vi "bob1tobun.vi"() -> ()   [LabVIEW 2014, in "Panels.lvlib"]
uses:
  Panels.lvlib
  CSlibraries-extern/DimLVEvent/DimIndicators/DimIndicators.lvlib
  CSlibraries/UtilityLib/UtilityLib.lvlib
  CS_Core/CSSystem/CoreLib/CoreLib.lvlib
  CSlibraries/UtilityLib/UtilityLib.valueStatus.ctl
  CSlibraries-extern/DimLVEvent/LVDimInterface/LVDimInterface.lvlib
  Instance           1 17Saved   bob1tobun .vi
  CSlibraries-extern/DimLVEvent/DimIndicators/DimIndicators.numericArrayType.ctl
  CSlibraries-extern/DimLVEvent/DimIndicators/DimIndicators.anyType.ctl
  CSlibraries-extern/DimLVEvent/DimIndicators/DimIndicators.numericType.ctl
panel:
  out "DIM Error":bool
  in  "SetFileLocation_Data":T1={"data"="NOLINK", "no link"=TRUE, "quality"=-1, "timeStamp"=0.0}
  in  "Q90PlanDefY":bool
  in  "ISDefY":bool
  in  "Q90PlanLens":bool
  in  "BOB3DefY":bool
  in  "BOB3DefX":bool
  in  "BOB2Q90Lens":bool
  in  "Q90DefMain":bool
  in  "Q90BOB3Lens":bool
  in  "ISDefX":bool
  in  "Q90CylLens":bool
  in  "BOB2DefX":bool
  in  "BOB2DefY":bool
  in  "WalLens":bool
  in  "BOB1DefX":bool
  in  "BOB1DefY":bool
  in  "Q90DefMain_MonData":T2={"data"=inf, "no link"=FALSE, "quality"=1, "timeStamp"=3265900746.554}
  in  "Q90BOB3Lens_MonData":T2={"data"=inf, "no link"=FALSE, "quality"=1, "timeStamp"=3265900746.538}
  in  "Q90PlanLens_MonData":T2={"data"=inf, "no link"=FALSE, "quality"=1, "timeStamp"=3265900746.522}
  in  "BOB3DefX_MonData":T2={"data"=inf, "no link"=FALSE, "quality"=1, "timeStamp"=3265900746.554}
  in  "BOB1DefX_MonData":T2={"data"=inf, "no link"=FALSE, "quality"=1, "timeStamp"=3265900746.538}
  in  "WalLens_MonData":T2={"data"=inf, "no link"=FALSE, "quality"=1, "timeStamp"=3265900746.569}
  in  "BOB2Q90Lens_MonData":T2={"data"=inf, "no link"=FALSE, "quality"=1, "timeStamp"=3265900746.554}
  in  "ISDefX_MonData":T2={"data"=inf, "no link"=FALSE, "quality"=1, "timeStamp"=3265900746.538}
  in  "BOB2DefX_MonData":T2={"data"=inf, "no link"=FALSE, "quality"=1, "timeStamp"=3265900746.569}
  in  "BOB3DefY_MonData":T2={"data"=inf, "no link"=FALSE, "quality"=1, "timeStamp"=3265900746.569}
  in  "Q90DefCorr1_MonData":T2={"data"=inf, "no link"=FALSE, "quality"=1, "timeStamp"=3265900746.538}
  in  "Q90DefCorr2_MonData":T2={"data"=inf, "no link"=FALSE, "quality"=1, "timeStamp"=3265900746.585}
  in  "Q90PlanDefY_MonData":T2={"data"=inf, "no link"=FALSE, "quality"=1, "timeStamp"=3265900746.538}
  in  "Q90DefMain1_MonData":T2={"data"=inf, "no link"=FALSE, "quality"=1, "timeStamp"=3265900746.554}
  in  "ISDefY_MonData":T2={"data"=inf, "no link"=FALSE, "quality"=1, "timeStamp"=3265900746.522}
  in  "BOB1DefY_MonData":T2={"data"=inf, "no link"=FALSE, "quality"=1, "timeStamp"=3265900746.538}
  in  "BOB2DefY_MonData":T2={"data"=inf, "no link"=FALSE, "quality"=1, "timeStamp"=3265900746.6}
  in  "Q90CylLens_MonData":T2={"data"=inf, "no link"=FALSE, "quality"=1, "timeStamp"=3265900746.585}
  in  "Q90DefMain2_MonData":T2={"data"=inf, "no link"=FALSE, "quality"=1, "timeStamp"=3265900746.569}
  in  "Q90DefMain_SetValueInfoData":T3={"data"=[-400.0, 400.0, 3.0], "no link"=FALSE, "quality"=0, "timeStamp"=3265900746.554}
  in  "Q90DefMain_SetData":T3={"data"=[0.0, 0.0, 0.0, 0.0], "no link"=FALSE, "quality"=1, "timeStamp"=3265900745.1}
  out "Q90DefMain_Mon":dbl=inf format="%.4f"
  in  "BOB1DefX_SetValueInfoData":T3={"data"=[-404.0, 401.8, 3.0], "no link"=FALSE, "quality"=0, "timeStamp"=3265900746.569}
  in  "BOB1DefX_SetData":T3={"data"=[0.0, 0.0, 0.0, 0.0], "no link"=FALSE, "quality"=1, "timeStamp"=3265900745.053}
  out "BOB3DefX_Mon":dbl=inf format="%.4f"
  in  "BOB1DefY_SetData":T3={"data"=[0.0, 0.0, 0.0, 0.0], "no link"=FALSE, "quality"=1, "timeStamp"=3265900745.053}
  in  "BOB3DefY_SetValueInfoData":T3={"data"=[-400.0, 400.0, 3.0], "no link"=FALSE, "quality"=0, "timeStamp"=3265900746.554}
  in  "BOB3DefX_SetValueInfoData":T3={"data"=[-400.0, 400.0, 3.0], "no link"=FALSE, "quality"=0, "timeStamp"=3265900746.538}
  in  "Q90BOB3Lens_SetValueInfoData":T3={"data"=[-400.0, 400.0, 3.0], "no link"=FALSE, "quality"=0, "timeStamp"=3265900746.522}
  in  "ISDefY_SetValueInfoData":T3={"data"=[-118.7, 118.8, 3.0], "no link"=FALSE, "quality"=0, "timeStamp"=3265900746.569}
  in  "Q90PlanDefY_SetValueInfoData":T3={"data"=[-120.9, 120.5, 3.0], "no link"=FALSE, "quality"=0, "timeStamp"=3265900746.585}
  in  "Q90PlanLens_SetValueInfoData":T3={"data"=[-120.8, 120.3, 3.0], "no link"=FALSE, "quality"=0, "timeStamp"=3265900746.569}
  in  "BOB3DefY_SetData":T3={"data"=[0.0, 0.0, 0.0, 0.0], "no link"=FALSE, "quality"=1, "timeStamp"=3265900745.1}
  in  "BOB3DefX_SetData":T3={"data"=[0.0, 0.0, 0.0, 0.0], "no link"=FALSE, "quality"=1, "timeStamp"=3265900745.085}
  in  "Q90BOB3Lens_SetData":T3={"data"=[0.0, 0.0, 0.0, 0.0], "no link"=FALSE, "quality"=1, "timeStamp"=3265900745.069}
  in  "ISDefY_SetData":T3={"data"=[0.0, 0.0, 0.0, 0.0], "no link"=FALSE, "quality"=1, "timeStamp"=3265900745.069}
  in  "Q90PlanDefY_SetData":T3={"data"=[0.0, 0.0, 0.0, 0.0], "no link"=FALSE, "quality"=1, "timeStamp"=3265900745.069}
  out "Q90PlanLens_Mon":dbl=inf format="%.4f"
  out "Q90BOB3Lens_Mon":dbl=inf format="%.4f"
  out "BOB3DefY_Mon":dbl=inf format="%.4f"
  out "Q90DefMain1_Mon":dbl=inf format="%.4f"
  out "Q90DefCorr2_Mon":dbl=inf format="%.4f"
  out "Q90DefCorr1_Mon":dbl=inf format="%.4f"
  out "Q90PlanDefY_Mon":dbl=inf format="%.4f"
  in  "Q90PlanLens_SetData":T3={"data"=[0.0, 0.0, 0.0, 0.0], "no link"=FALSE, "quality"=1, "timeStamp"=3265900745.069}
  out "WalLens_Mon":dbl=inf format="%.4f"
  out "BOB1DefX_Mon":dbl=inf format="%.4f"
  out "i ref out":refnum<vi>
  in  "Last Loaded File_Data":T1={"data"="NOLINK", "no link"=TRUE, "quality"=-1, "timeStamp"=0.0}
  out "FileUpToDate":bool=TRUE caption="Parameter Changed"
  in  "Close All Panels":bool
  in  "WalLens_SetValueInfoData":T3={"data"=[-401.3, 400.4, 3.0], "no link"=FALSE, "quality"=0, "timeStamp"=3265900746.554}
  in  "BOB2Q90Lens_SetValueInfoData":T3={"data"=[-404.3, 403.0, 3.0], "no link"=FALSE, "quality"=0, "timeStamp"=3265900746.538}
  in  "BOB2DefX_SetValueInfoData":T3={"data"=[-400.3, 399.3, 3.0], "no link"=FALSE, "quality"=0, "timeStamp"=3265900746.569}
  in  "BOB2DefY_SetValueInfoData":T3={"data"=[0.0, 3000.0, -1.0], "no link"=FALSE, "quality"=0, "timeStamp"=3265900746.554}
  in  "Q90CylLens_SetValueInfoData":T3={"data"=[0.0, 1500.0, -1.0], "no link"=FALSE, "quality"=0, "timeStamp"=3265900746.554}
  in  "ISDefX_SetValueInfoData":T3={"data"=[0.0, 1000.0, -1.0], "no link"=FALSE, "quality"=0, "timeStamp"=3265900746.538}
  in  "BOB1DefY_SetValueInfoData":T3={"data"=[-404.0, 401.8, 3.0], "no link"=FALSE, "quality"=0, "timeStamp"=3265900746.569}
  in  "ISDefX_SetData":T3={"data"=[0.0, 0.0, 0.0, 0.0], "no link"=FALSE, "quality"=1, "timeStamp"=3265900745.069}
  in  "Q90CylLens_SetData":T3={"data"=[0.0, 0.0, 0.0, 0.0], "no link"=FALSE, "quality"=1, "timeStamp"=3265900745.053}
  in  "BOB2DefY_SetData":T3={"data"=[0.0, 0.0, 0.0, 0.0], "no link"=FALSE, "quality"=1, "timeStamp"=3265900745.085}
  in  "BOB2DefX_SetData":T3={"data"=[0.0, 0.0, 0.0, 0.0], "no link"=FALSE, "quality"=1, "timeStamp"=3265900745.085}
  in  "BOB2Q90Lens_SetData":T3={"data"=[0.0, 0.0, 0.0, 0.0], "no link"=FALSE, "quality"=1, "timeStamp"=3265900745.085}
  in  "WalLens_SetData":T3={"data"=[0.0, 0.0, 0.0, 0.0], "no link"=FALSE, "quality"=1, "timeStamp"=3265900745.053}
  out "Last Loaded File":string
  in  "SetFileLocation":path=path "\\\\intranet\\Files/projects/lebit/Data Exchange/data/bob1tobunControl"
  out "ISDefY_Mon":dbl=inf format="%.4f"
  out "Q90CylLens_Mon":dbl=inf format="%.4f"
  out "BOB1DefY_Mon":dbl=inf format="%.4f"
  out "BOB2DefY_Mon":dbl=inf format="%.4f"
  out "Q90DefMain2_Mon":dbl=inf format="%.4f"
  out "BOB2DefX_Mon":dbl=inf format="%.4f"
  out "ISDefX_Mon":dbl=inf format="%.4f"
  out "BOB2Q90Lens_Mon":dbl=inf format="%.4f"
  # "Parameter changed, data file is no longer up-to-date."
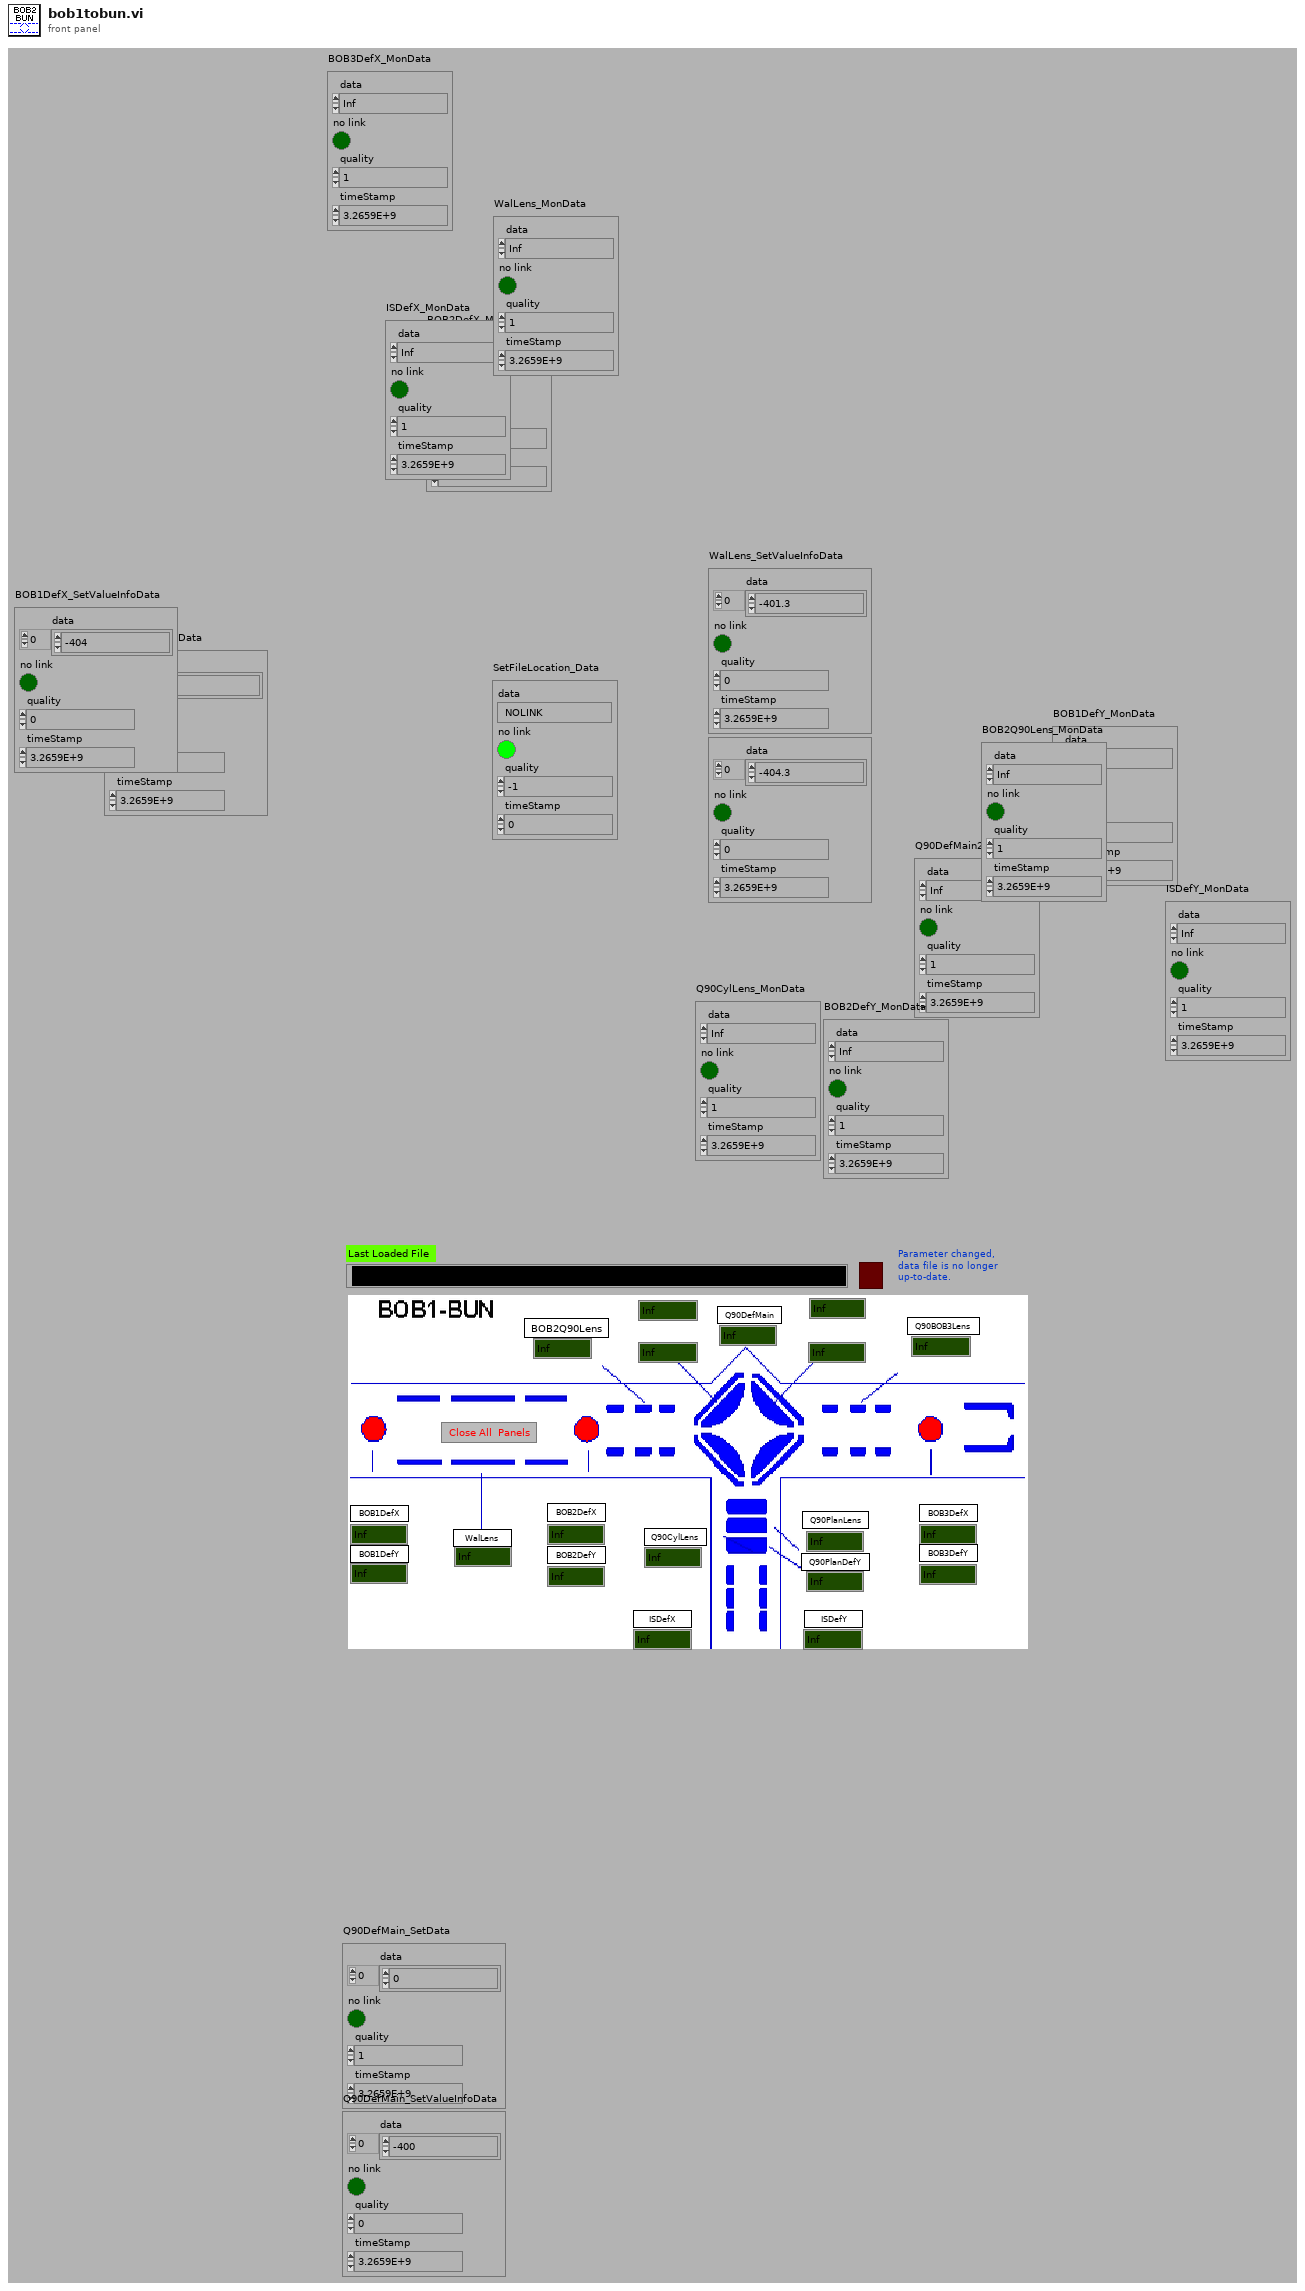
[diagram p1: front panel]
types:
  T1 = typedef "DimIndicators.lvlib/DimIndicators.anyType.ctl" = cluster{"data":string, "no link":bool, "quality":i32, "timeStamp":dbl}
  T2 = typedef "DimIndicators.lvlib/DimIndicators.numericType.ctl" = cluster{"data":dbl, "no link":bool, "quality":i32, "timeStamp":dbl}
  T3 = typedef "DimIndicators.lvlib/DimIndicators.numericArrayType.ctl" = cluster{"data":dbl[], "no link":bool, "quality":i32, "timeStamp":dbl}
  T4 = typedef "UtilityLib.lvlib/UtilityLib.valueStatus.ctl" = enum16{"no info available", "stand by/off", "on", "warning", "alarm/malfunction", "not implemented", "user action required", "important information", "system default", "control default", "indicator default", "button default"}
  T5 = cluster{"data":string, "no link":bool, "quality":i32, "timeStamp":dbl}
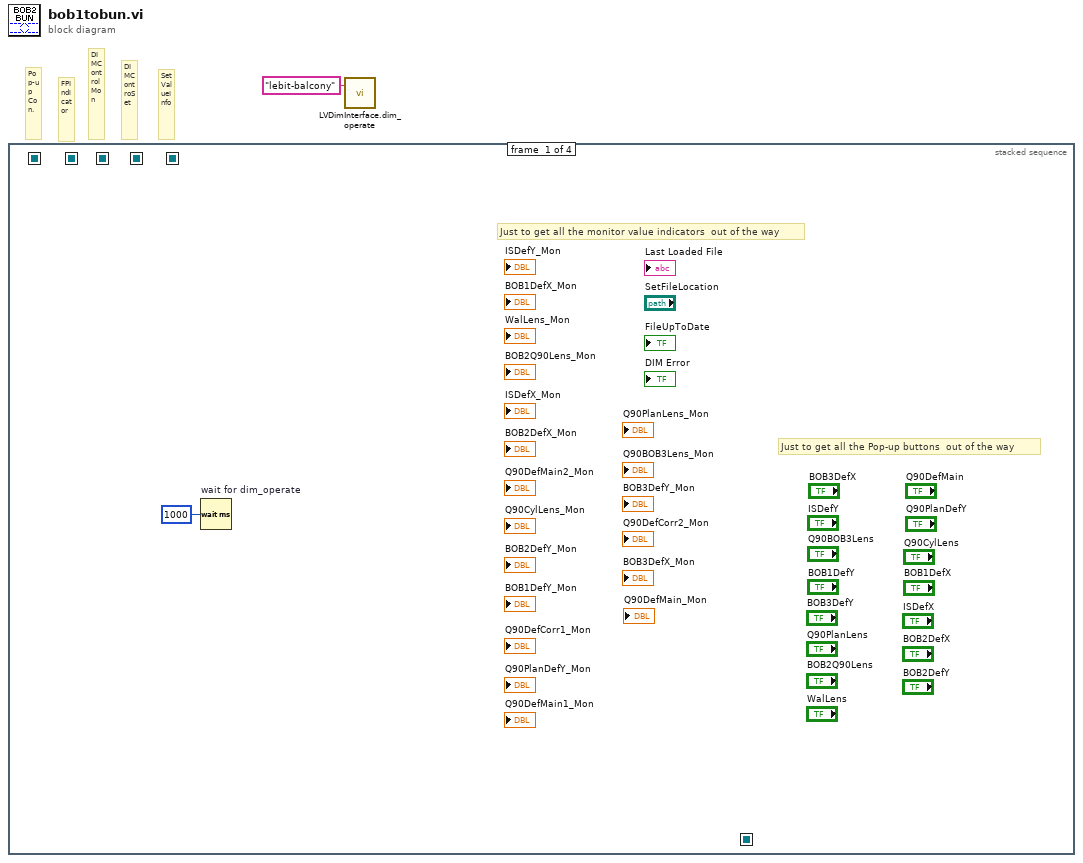
[diagram p0: block diagram]
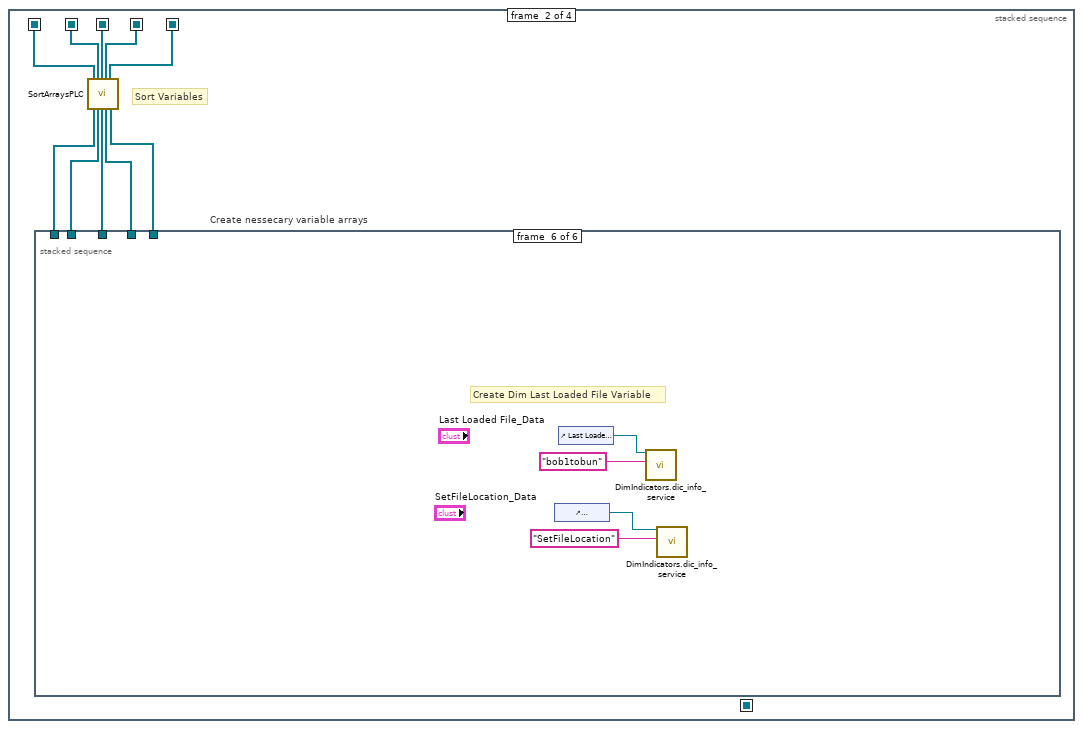
[diagram p2: hidden frame]
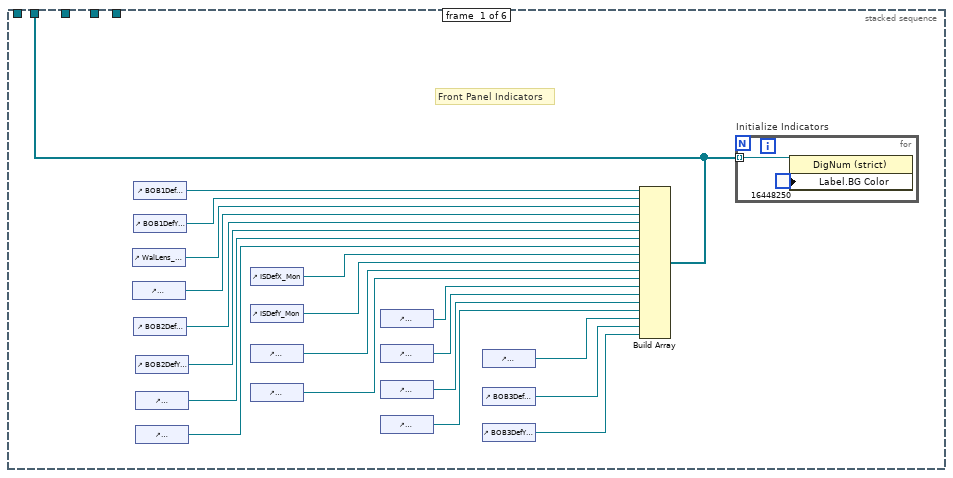
[diagram p3: hidden frame]
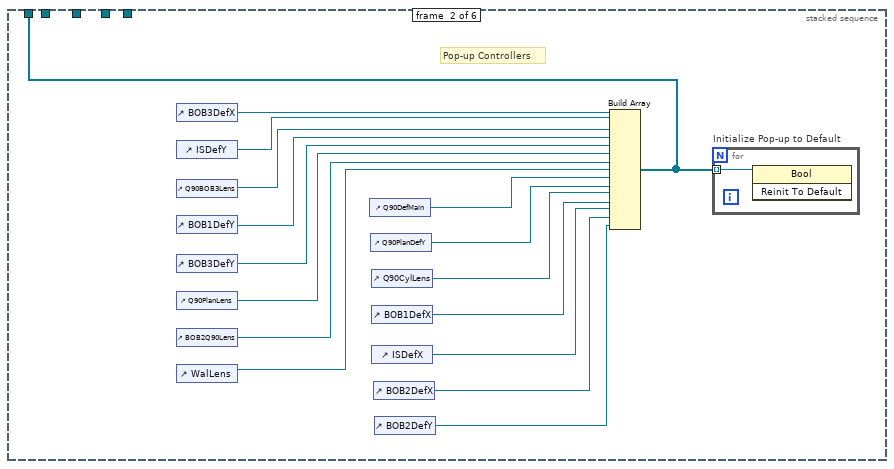
[diagram p4: hidden frame]
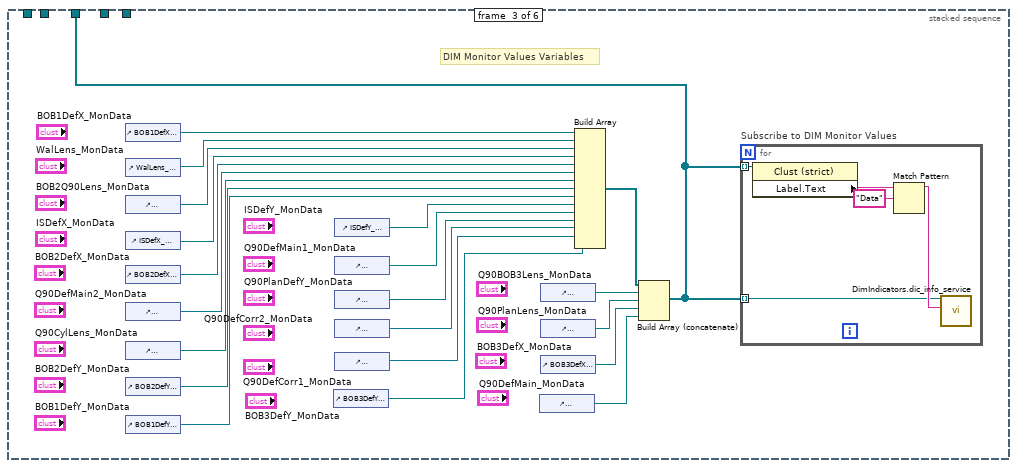
[diagram p5: hidden frame]
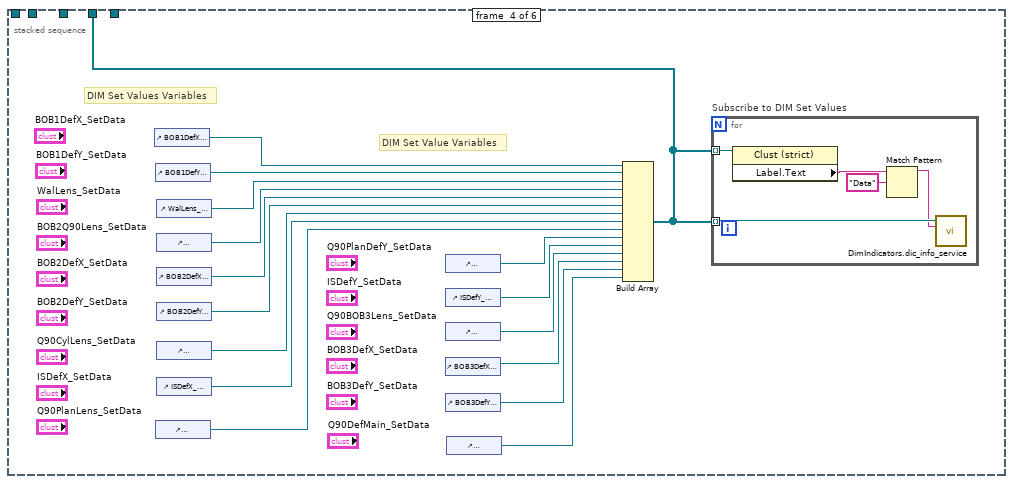
[diagram p6: hidden frame]
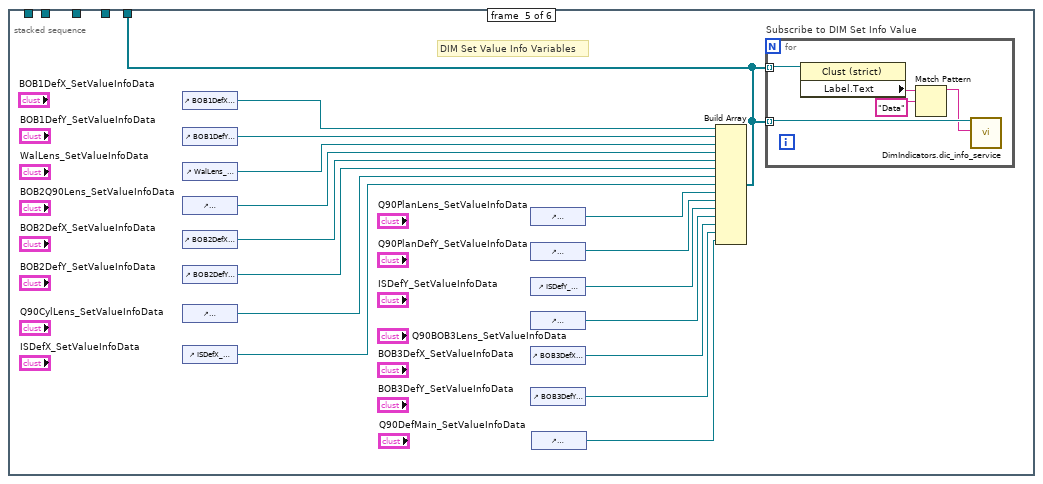
[diagram p7: hidden frame]
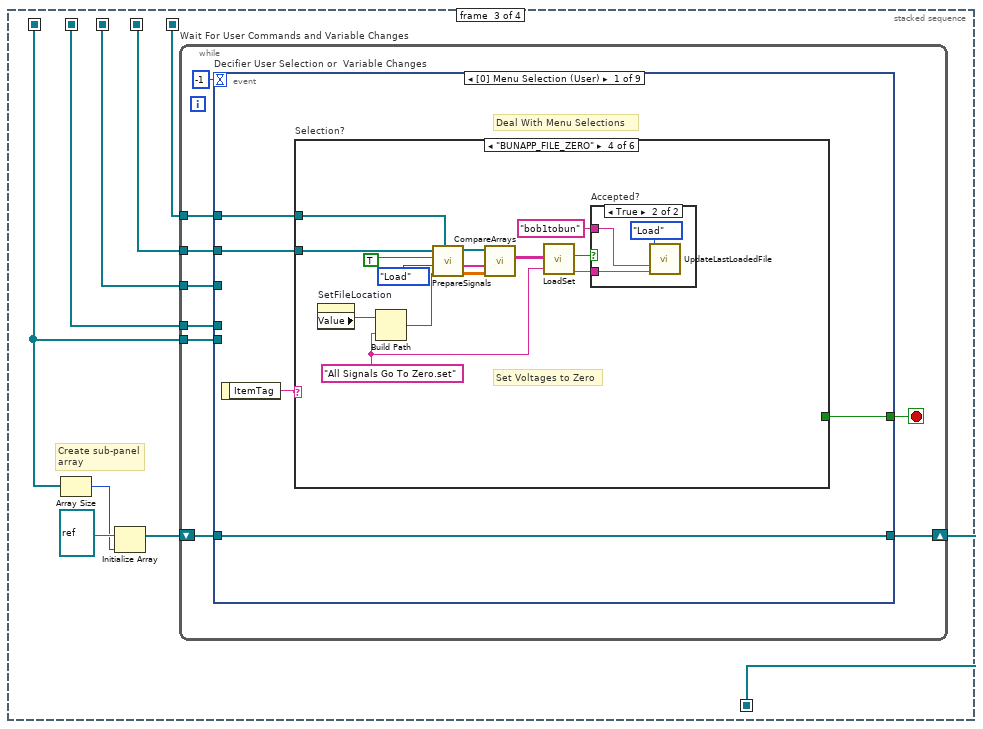
[diagram p8: hidden frame]
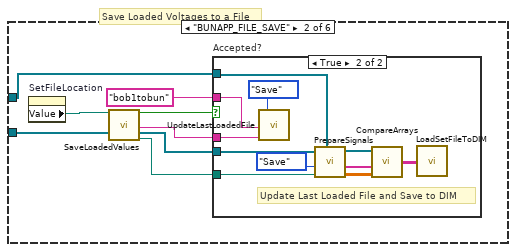
[diagram p10: hidden frame]
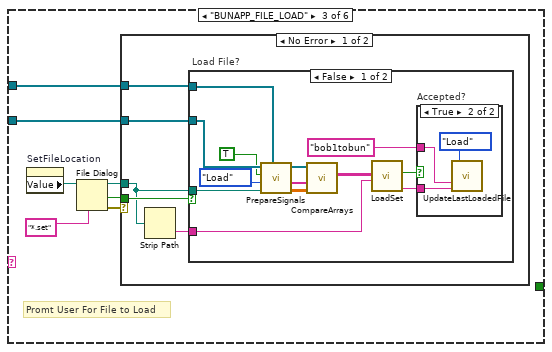
[diagram p12: hidden frame]
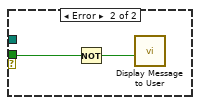
[diagram p15: hidden frame]
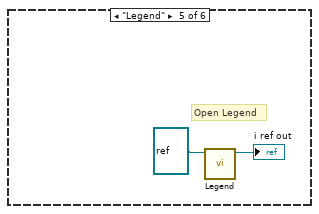
[diagram p17: hidden frame]
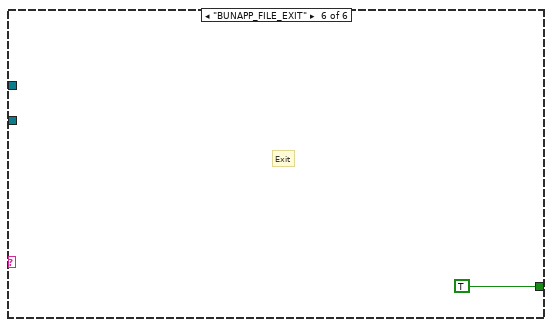
[diagram p18: hidden frame]
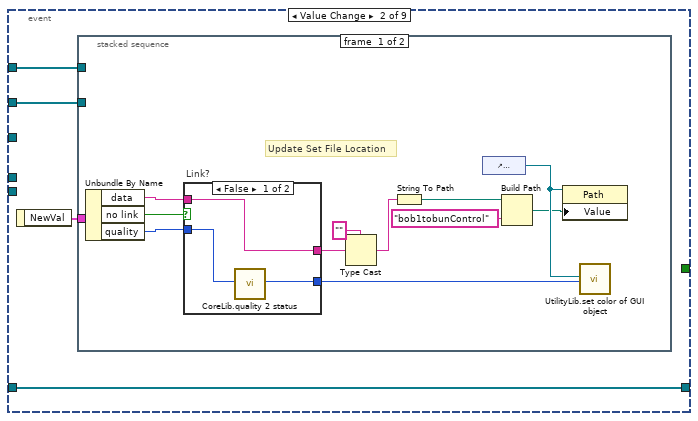
[diagram p19: hidden frame]
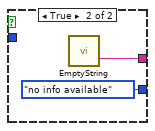
[diagram p20: hidden frame]
diagram:
  # "Pop-up Con."
  # "SetValueInfo"
  # "DIMControSet"
  # "DIMControlMon"
  # "FPIndicator"
  n1 = stacked-sequence {
    seq-local: [_ w4 _ _] -> [_ _ w130 _]
    seq-local: [_ w5 _ _] -> [_ _ w125 w325]
    seq-local: [_ _ w128 _] -> [_ _ _ w324]
    seq-local: [_ w6 _ _] -> [_ _ w127 w323]
    seq-local: [_ w7 _ _] -> [_ _ w126 w322]
    seq-local: [_ w3 _ _] -> [_ _ w124 _]
    frame #0 {
      # "Just to get all the Pop-up buttons  out of the way"
      # "Just to get all the monitor value indicators  out of the way"
      n2 = Wait (ms) "wait for dim_operate"(milliseconds to wait=u32 1000) -> ()  [unwired: 1 out]
    }
    frame #1 {
      # "Sort Variables"
      # "Arrange references to all monitor-value related buttons into an array."
      n3 = stacked-sequence "Create nessecary variable arrays" {
        tunnel: [w31 _ _ _ _ _] -> w11
        tunnel: [_ w35 _ _ _ _] -> w12
        tunnel: [_ _ w52 _ _ _] -> w10
        tunnel: [_ _ _ w78 _ _] -> w9
        tunnel: [_ _ _ _ w99 _] -> w8
        frame #0 {
          # "Front Panel Indicators"
          n4 = control-ref of="WalLens_Mon"() -> (w24:refnum<vi>)
          n5 = control-ref of="BOB2Q90Lens_Mon"() -> (w23:refnum<vi>)
          n6 = control-ref of="BOB1DefX_Mon"() -> (w30:refnum<vi>)
          n7 = control-ref of="BOB1DefY_Mon"() -> (w25:refnum<vi>)
          n8 = control-ref of="BOB2DefX_Mon"() -> (w32:refnum<vi>)
          n9 = control-ref of="BOB2DefY_Mon"() -> (w21:refnum<vi>)
          n10 = control-ref of="Q90DefMain2_Mon"() -> (w20:refnum<vi>)
          n11 = control-ref of="Q90CylLens_Mon"() -> (w19:refnum<vi>)
          n12 = control-ref of="ISDefX_Mon"() -> (w22:refnum<vi>)
          n13 = control-ref of="ISDefY_Mon"() -> (w29:refnum<vi>)
          n14 = control-ref of="Q90DefMain_Mon"() -> (w17:refnum<vi>)
          n15 = control-ref of="Q90DefMain1_Mon"() -> (w16:refnum<vi>)
          n16 = control-ref of="Q90DefCorr2_Mon"() -> (w28:refnum<vi>)
          n17 = control-ref of="Q90DefCorr1_Mon"() -> (w27:refnum<vi>)
          n18 = control-ref of="Q90PlanLens_Mon"() -> (w15:refnum<vi>)
          n19 = control-ref of="Q90PlanDefY_Mon"() -> (w14:refnum<vi>)
          n20 = control-ref of="Q90BOB3Lens_Mon"() -> (w13:refnum<vi>)
          n21 = control-ref of="BOB3DefX_Mon"() -> (w26:refnum<vi>)
          n22 = control-ref of="BOB3DefY_Mon"() -> (w18:refnum<vi>)
          n23 = Build Array(w30, w25, w24, w23, w32, w21, w20, w19, w22, w29, w17, w16, w28, w27, w15, w14, w13, w26, w18) -> (w31:refnum<vi>[])
          n24 = for "Initialize Indicators" {
            tunnel: w31 -> [w34] mode=indexing
            n25 = property class="DigNum (strict)"(reference=w34, "Label.BG Color"=u32 16448250 ("Color Box")) -> ()  [unwired: 1 in, 2 out]
          }
        }
        frame #1 {
          # "Pop-up Controllers"
          n26 = control-ref of="BOB3DefX"() -> (w50:refnum<vi>)
          n27 = control-ref of="ISDefY"() -> (w49:refnum<vi>)
          n28 = control-ref of="Q90BOB3Lens"() -> (w48:refnum<vi>)
          n29 = control-ref of="BOB1DefY"() -> (w47:refnum<vi>)
          n30 = control-ref of="BOB3DefY"() -> (w46:refnum<vi>)
          n31 = control-ref of="Q90PlanLens"() -> (w45:refnum<vi>)
          n32 = control-ref of="BOB2Q90Lens"() -> (w44:refnum<vi>)
          n33 = control-ref of="WalLens"() -> (w43:refnum<vi>)
          n34 = control-ref of="Q90DefMain"() -> (w42:refnum<vi>)
          n35 = control-ref of="Q90PlanDefY"() -> (w41:refnum<vi>)
          n36 = control-ref of="Q90CylLens"() -> (w40:refnum<vi>)
          n37 = control-ref of="BOB1DefX"() -> (w39:refnum<vi>)
          n38 = control-ref of="ISDefX"() -> (w38:refnum<vi>)
          n39 = control-ref of="BOB2DefX"() -> (w37:refnum<vi>)
          n40 = control-ref of="BOB2DefY"() -> (w36:refnum<vi>)
          n41 = Build Array(w50, w49, w48, w47, w46, w45, w44, w43, w42, w41, w40, w39, w38, w37, w36) -> (w35:refnum<vi>[])
          n42 = for "Initialize Pop-up to Default" {
            tunnel: w35 -> [w51] mode=indexing
            n43 = invoke class="Bool" method="Reinit To Default"(reference=w51) -> ()  [unwired: 2 in, 3 out]
          }
        }
        frame #2 {
          # "DIM Monitor Values Variables"
          n44 = control-ref of="BOB1DefX_MonData"() -> (w68:refnum<vi>)
          n45 = control-ref of="WalLens_MonData"() -> (w67:refnum<vi>)
          n46 = control-ref of="BOB2Q90Lens_MonData"() -> (w66:refnum<vi>)
          n47 = control-ref of="ISDefX_MonData"() -> (w61:refnum<vi>)
          n48 = control-ref of="BOB2DefX_MonData"() -> (w62:refnum<vi>)
          n49 = control-ref of="Q90DefMain2_MonData"() -> (w54:refnum<vi>)
          n50 = control-ref of="Q90CylLens_MonData"() -> (w55:refnum<vi>)
          n51 = control-ref of="BOB2DefY_MonData"() -> (w56:refnum<vi>)
          n52 = control-ref of="BOB1DefY_MonData"() -> (w57:refnum<vi>)
          n53 = control-ref of="BOB3DefY_MonData"() -> (w53:refnum<vi>)
          n54 = control-ref of="ISDefY_MonData"() -> (w58:refnum<vi>)
          n55 = control-ref of="Q90DefMain1_MonData"() -> (w59:refnum<vi>)
          n56 = control-ref of="Q90PlanDefY_MonData"() -> (w60:refnum<vi>)
          n57 = control-ref of="Q90DefCorr2_MonData"() -> (w69:refnum<vi>)
          n58 = control-ref of="Q90DefCorr1_MonData"() -> (w70:refnum<vi>)
          n59 = control-ref of="Q90DefMain_MonData"() -> (w72:refnum<vi>)
          n60 = control-ref of="Q90BOB3Lens_MonData"() -> (w63:refnum<vi>)
          n61 = control-ref of="Q90PlanLens_MonData"() -> (w64:refnum<vi>)
          n62 = control-ref of="BOB3DefX_MonData"() -> (w65:refnum<vi>)
          n63 = Build Array(w68, w67, w66, w61, w62, w54, w55, w56, w57, w58, w59, w60, w69, w70, w53) -> (w71:refnum<vi>[])
          n64 = Build Array (concatenate)(w71, w63, w64, w65, w72) -> (w52:refnum<vi>[])
          n65 = for "Subscribe to DIM Monitor Values" {
            tunnel: w52 -> [w74] mode=indexing
            tunnel: w52 -> [w73] mode=indexing
            n66 = property class="Clust (strict)"(reference=w73) -> ("Label.Text"=w76:string)  [unwired: 1 in, 2 out]
            n67 = Match Pattern(string=w76, regular expression="Data") -> (before substring=w75:string)  [unwired: 1 in, 3 out]
            n68 = call "DimIndicators.dic_info_service.vi"("controlRef"=w74, "serviceName"=w75) -> ()  [unwired: 16 in, 2 out]
          }
        }
        frame #3 {
          # "DIM Set Value Variables"
          # "DIM Set Values Variables"
          n69 = control-ref of="BOB1DefX_SetData"() -> (w80:refnum<vi>)
          n70 = control-ref of="BOB1DefY_SetData"() -> (w81:refnum<vi>)
          n71 = control-ref of="Q90PlanLens_SetData"() -> (w87:refnum<vi>)
          n72 = control-ref of="WalLens_SetData"() -> (w93:refnum<vi>)
          n73 = control-ref of="BOB2Q90Lens_SetData"() -> (w92:refnum<vi>)
          n74 = control-ref of="BOB2DefX_SetData"() -> (w91:refnum<vi>)
          n75 = control-ref of="BOB2DefY_SetData"() -> (w90:refnum<vi>)
          n76 = control-ref of="Q90CylLens_SetData"() -> (w89:refnum<vi>)
          n77 = control-ref of="ISDefX_SetData"() -> (w88:refnum<vi>)
          n78 = control-ref of="Q90PlanDefY_SetData"() -> (w86:refnum<vi>)
          n79 = control-ref of="ISDefY_SetData"() -> (w85:refnum<vi>)
          n80 = control-ref of="Q90BOB3Lens_SetData"() -> (w84:refnum<vi>)
          n81 = control-ref of="BOB3DefX_SetData"() -> (w83:refnum<vi>)
          n82 = control-ref of="BOB3DefY_SetData"() -> (w82:refnum<vi>)
          n83 = control-ref of="Q90DefMain_SetData"() -> (w79:refnum<vi>)
          n84 = Build Array(w80, w81, w93, w92, w91, w90, w89, w88, w87, w86, w85, w84, w83, w82, w79) -> (w78:refnum<vi>[])
          n85 = for "Subscribe to DIM Set Values" {
            tunnel: w78 -> [w94] mode=indexing
            tunnel: w78 -> [w98] mode=indexing
            n86 = property class="Clust (strict)"(reference=w94) -> ("Label.Text"=w97:string)  [unwired: 1 in, 2 out]
            n87 = Match Pattern(string=w97, regular expression="Data") -> (before substring=w95:string)  [unwired: 1 in, 3 out]
            n88 = call "DimIndicators.dic_info_service.vi"("controlRef"=w98, "serviceName"=w95) -> ()  [unwired: 16 in, 2 out]
          }
        }
        frame #4 {
          # "DIM Set Value Info Variables"
          n89 = control-ref of="BOB1DefX_SetValueInfoData"() -> (w101:refnum<vi>)
          n90 = control-ref of="BOB1DefY_SetValueInfoData"() -> (w114:refnum<vi>)
          n91 = control-ref of="WalLens_SetValueInfoData"() -> (w113:refnum<vi>)
          n92 = control-ref of="BOB2Q90Lens_SetValueInfoData"() -> (w112:refnum<vi>)
          n93 = control-ref of="BOB2DefX_SetValueInfoData"() -> (w111:refnum<vi>)
          n94 = control-ref of="BOB2DefY_SetValueInfoData"() -> (w110:refnum<vi>)
          n95 = control-ref of="Q90CylLens_SetValueInfoData"() -> (w109:refnum<vi>)
          n96 = control-ref of="ISDefX_SetValueInfoData"() -> (w108:refnum<vi>)
          n97 = control-ref of="Q90PlanLens_SetValueInfoData"() -> (w107:refnum<vi>)
          n98 = control-ref of="Q90PlanDefY_SetValueInfoData"() -> (w106:refnum<vi>)
          n99 = control-ref of="ISDefY_SetValueInfoData"() -> (w105:refnum<vi>)
          n100 = control-ref of="Q90BOB3Lens_SetValueInfoData"() -> (w104:refnum<vi>)
          n101 = control-ref of="BOB3DefX_SetValueInfoData"() -> (w103:refnum<vi>)
          n102 = control-ref of="BOB3DefY_SetValueInfoData"() -> (w102:refnum<vi>)
          n103 = control-ref of="Q90DefMain_SetValueInfoData"() -> (w100:refnum<vi>)
          n104 = Build Array(w101, w114, w113, w112, w111, w110, w109, w108, w107, w106, w105, w104, w103, w102, w100) -> (w99:refnum<vi>[])
          n105 = for "Subscribe to DIM Set Info Value" {
            tunnel: w99 -> [w115] mode=indexing
            tunnel: w99 -> [w119] mode=indexing
            n106 = property class="Clust (strict)"(reference=w115) -> ("Label.Text"=w118:string)  [unwired: 1 in, 2 out]
            n107 = Match Pattern(string=w118, regular expression="Data") -> (before substring=w116:string)  [unwired: 1 in, 3 out]
            n108 = call "DimIndicators.dic_info_service.vi"("controlRef"=w119, "serviceName"=w116) -> ()  [unwired: 16 in, 2 out]
          }
        }
        frame #5 {
          # "Create Dim Last Loaded File Variable"
          n109 = control-ref of="SetFileLocation_Data"() -> (w123:refnum<vi>)
          n110 = control-ref of="Last Loaded File_Data"() -> (w121:refnum<vi>)
          n111 = call "DimIndicators.dic_info_service.vi"("controlRef"=w121, "serviceName"="bob1tobun" ("string")) -> ()  [unwired: 16 in, 2 out]
          n112 = call "DimIndicators.dic_info_service.vi"("controlRef"=w123, "serviceName"="SetFileLocation" ("string")) -> ()  [unwired: 16 in, 2 out]
        }
      }
      n113 = call "SortArraysPLC.vi"("Pop-up Con."=w12, "FPIndicator in"=w11, "DIMControlMon"=w10, "DIMControSet"=w9, "SetValueInfo"=w8) -> ("Pop-up Con. out"=w3:refnum<vi>[], "FPIndicator out"=w4:refnum<vi>[], "DIMControlMon out"=w5:refnum<vi>[], "DIMControSet out"=w6:refnum<vi>[], "SetValueInfo out"=w7:refnum<vi>[])  [unwired: 18 in]
    }
    frame #2 {
      # "Create sub-panel\narray"
      n114 = Array Size(array=w124) -> (size(s)=w129:i32)
      n115 = Initialize Array(refnum<vi> refnum ("vi reference"), w129) -> (w132:refnum<vi>[])
      n116 = while "Wait For User Commands and Variable Changes" {
        tunnel: w130 -> [w141]
        shift-right: [w139] -> w128
        shift-left: w132 -> [w140]
        tunnel: w127 -> [w138]
        tunnel: w126 -> [w137]
        tunnel: w125 -> [w135]
        tunnel: w124 -> [w134]
        stop <- w133 stop-if-true
        n117 = event "Decifier User Selection or  Variable Changes" shown="[0] Menu Selection (User)" {
          selector: _ -> [_ _ _ _ _ _ _ _ _]
          dyn-events: _ -> [_ _ _ _ _ _ _ _ _]
          timeout: -1 -> [_ _ _ _ _ _ _ _ _]
          tunnel: [w143 _ _ _ _ _ _ _ TRUE ("stop")] -> w133
          tunnel: w141 -> [_ _ _ w253 _ _ _ _ _]
          tunnel: w140 -> [w146 w218 w250 w257 w275 w283 w290 w296 w300]
          tunnel: [w146 w218 w250 w257 w275 w281 w288 w296 _] -> w139
          tunnel: w138 -> [w144 w217 w245 _ w273 _ _ _ w298]
          tunnel: w137 -> [w142 w216 w244 _ _ _ _ _ w299]
          tunnel: w135 -> [_ _ _ w256 _ _ _ _ w297]
          tunnel: w134 -> [_ _ _ _ _ w276 _ _ _]
          event Menu Selection (User) {
            # "Deal With Menu Selections"
            n118 = event-data() -> ("ItemTag"=w145:string)  [unwired: 1 in]
            n119 = case "Selection?" shown="\"BUNAPP_FILE_ZERO\"" w145 {
              tunnel: w144 -> [_ w151 w171 w209 _ _]
              tunnel: [_ _ _ _ _ TRUE ("stop")] -> w143
              tunnel: w142 -> [_ w147 w166 w196 _ _]
              frame "False", Default {
              }
              frame "BUNAPP_FILE_SAVE" {
                # "Save Loaded Voltages to a File"
                n120 = property on="SetFileLocation" class="Path"() -> ("Value"=w152:path)  [unwired: 2 in, 2 out]
                n121 = call "SaveLoadedValues.vi"("Panel Location?"=w152, "DIMControlSet in"=w151) -> ("File Saved?"=w153:bool, "File Name"=w150:string, "DIMControlSet out"=w148:refnum<vi>[], "Path"=w149:path)  [unwired: 14 in]
                n122 = case "Accepted?" shown="True" w153 {
                  tunnel: w150 -> [_ w163]
                  tunnel: "bob1tobun" ("string") -> [_ w165]
                  tunnel: w148 -> [_ w164]
                  tunnel: w149 -> [_ w162]
                  tunnel: w147 -> [_ w156]
                  frame False {
                  }
                  frame True {
                    # "Update Last Loaded File and Save to DIM"
                    n123 = call "UpdateLastLoadedFile.vi"("LoadOrSave"=enum16{"Load", "Save"}."Save", "GUIName"=w165, "FileNameIn"=w163) -> ()  [unwired: 13 in]
                    n124 = call "PrepareSignals.vi"("SetValueInfo in"=w156, "setfile path"=w162, "Enum"=enum16{"Save", "Load"}."Save", "DIMControSet in"=w164) -> ("indexed loaded Array"=w160:dbl[][], "Name Array"=w161:string[], "DIMControSet out"=w159:refnum<vi>[])  [unwired: 5 in]
                    n125 = call "CompareArrays.vi"("indexed loaded Array"=w160, "Name Array"=w161, "DIMControSet"=w159) -> ("Table for loading values"=w158:string[][])  [unwired: 4 in]
                    n126 = call "LoadSetFileToDIM.vi"("output array"=w158) -> ()  [unwired: 2 in]
                  }
                }
              }
              frame "BUNAPP_FILE_LOAD" {
                # "Promt User For File to Load"
                n127 = property on="SetFileLocation" class="Path"() -> ("Value"=w168:path)  [unwired: 2 in, 2 out]
                n128 = File Dialog(6:"*.set" ("pattern (all files)"), 11:w168) -> (0:w167:errorcluster, 1:w172:bool, 3:w169:path)  [unwired: 5 in, 1 out]
                n129 = case shown="No Error" w167 {
                  tunnel: w172 -> [w177 w194]
                  tunnel: w171 -> [w176 _]
                  tunnel: w169 -> [w174 _]
                  tunnel: w166 -> [w173 _]
                  frame No Error {
                    n130 = Strip Path(path=w174) -> (name=w175:string)  [unwired: 1 out]
                    n131 = case "Load File?" shown="False" w177 {
                      tunnel: w176 -> [w190 _]
                      tunnel: w175 -> [w184 _]
                      tunnel: w174 -> [w185 _]
                      tunnel: w173 -> [w178 _]
                      frame False {
                        n132 = call "PrepareSignals.vi"("SetValueInfo in"=w178, "setfile path"=w185, "Enum"=enum16{"Save", "Load"}."Load", "Display Message to \nUser"=TRUE ("Display Message to \nUser"), "DIMControSet in"=w190) -> ("indexed loaded Array"=w188:dbl[][], "Name Array"=w187:string[], "DIMControSet out"=w189:refnum<vi>[])  [unwired: 4 in]
                        n133 = call "CompareArrays.vi"("indexed loaded Array"=w188, "Name Array"=w187, "DIMControSet"=w189) -> ("Table for loading values"=w186:string[][])  [unwired: 4 in]
                        n134 = call "LoadSet.vi"("File Name In"=w184, "output array"=w186) -> ("File Name out"=w183:string, "Accepted"=w182:bool)  [unwired: 8 in]
                        n135 = case "Accepted?" shown="True" w182 {
                          tunnel: w183 -> [_ w193]
                          tunnel: "bob1tobun" ("string") -> [_ w192]
                          frame False {
                          }
                          frame True {
                            n136 = call "UpdateLastLoadedFile.vi"("LoadOrSave"=enum16{"Load", "Save"}."Load", "GUIName"=w192, "FileNameIn"=w193) -> ()  [unwired: 13 in]
                          }
                        }
                      }
                      frame True {
                      }
                    }
                  }
                  frame Error {
                    n137 = Not(x=w194) -> (.not. x?=w195:bool)
                    n138 = call "Display Message to User"("Enable"=w195) -> ()  [unwired: 9 in, 2 out]
                  }
                }
              }
              frame "BUNAPP_FILE_ZERO" {
                w200 = "All Signals Go To Zero.set" ("File Name")
                # "Set Voltages to Zero"
                n139 = property on="SetFileLocation" class="Path"() -> ("Value"=w198:path)  [unwired: 2 in, 2 out]
                n140 = Build Path(base path=w198, name or relative path=w200) -> (appended path=w199:path)
                n141 = call "PrepareSignals.vi"("SetValueInfo in"=w196, "setfile path"=w199, "Enum"=enum16{"Save", "Load"}."Load", "Display Message to \nUser"=TRUE ("Display Message to \nUser"), "DIMControSet in"=w209) -> ("indexed loaded Array"=w207:dbl[][], "Name Array"=w206:string[], "DIMControSet out"=w208:refnum<vi>[])  [unwired: 4 in]
                n142 = call "CompareArrays.vi"("indexed loaded Array"=w207, "Name Array"=w206, "DIMControSet"=w208) -> ("Table for loading values"=w205:string[][])  [unwired: 4 in]
                n143 = call "LoadSet.vi"("File Name In"=w200, "output array"=w205) -> ("File Name out"=w203:string, "Accepted"=w204:bool)  [unwired: 8 in]
                n144 = case "Accepted?" shown="True" w204 {
                  tunnel: w203 -> [_ w212]
                  tunnel: "bob1tobun" ("string") -> [_ w211]
                  frame False {
                  }
                  frame True {
                    n145 = call "UpdateLastLoadedFile.vi"("LoadOrSave"=enum16{"Load", "Save"}."Load", "GUIName"=w211, "FileNameIn"=w212) -> ()  [unwired: 13 in]
                  }
                }
              }
              frame "Legend" {
                # "Open Legend"
                n146 = call "Legend.vi"("i ref in"=refnum<vi> refnum) -> ("i ref out"=→"i ref out":refnum<vi>)  [unwired: 10 in]
              }
              frame "BUNAPP_FILE_EXIT" {
                # "Exit"
              }
            }
          }
          event Value Change {
            n147 = event-data() -> ("NewVal"=w219:T1)  [unwired: 1 in]
            n148 = stacked-sequence {
              tunnel: w219 -> [w225 _]
              tunnel: w217 -> [_ w243]
              tunnel: w216 -> [_ w237]
              frame #0 {
                # "Update Set File Location"
                n149 = Unbundle By Name(w225) -> ("data"=w230:string, "no link"=w229:bool, "quality"=w228:i32)
                n150 = case "Link?" shown="False" w229 {
                  tunnel: w228 -> [w234 _]
                  tunnel: [w233 UtilityLib.valueStatus."no info available" ("valueStatus")] -> w231
                  tunnel: w230 -> [w232 _]
                  tunnel: [w232 w235] -> w226
                  frame False {
                    n151 = call "CoreLib.quality 2 status.vi"("quality"=w234) -> ("valueStatus"=w233:T4)  [unwired: 18 in]
                  }
                  frame True {
                    n152 = call "EmptyString.vi"() -> ("String"=w235:string)
                  }
                }
                n153 = Type Cast(type="" ("regular expression"), x=w226) -> (*(type *) &x=w224:string)
                n154 = String To Path(string=w224) -> (path=w220:path)
                n155 = control-ref of="SetFileLocation"() -> (w222:refnum<vi>)
                n156 = Build Path(base path=w220, name or relative path="bob1tobunControl") -> (appended path=w221:path)
                n157 = property class="Path"(reference=w222, "Value"=w221) -> ()  [unwired: 1 in, 2 out]
                n158 = call "UtilityLib.set color of GUI object.vi"("GUI object Ref"=w222, "valueStatus"=w231) -> ()  [unwired: 17 in, 1 out]
              }
              frame #1 {
                # "Update Last Loaded File"
                n159 = control-ref of="SetFileLocation"() -> (w241:refnum<vi>)
                n160 = control-ref of="Last Loaded File"() -> (w242:refnum<vi>)
                n161 = control-ref of="Last Loaded File_Data"() -> (w240:refnum<vi>)
                n162 = property class="Clust (strict)"(reference=w240) -> ("Value"=w239:T5)  [unwired: 1 in, 2 out]
                n163 = call "LastLoadedFile.vi"("SetFileLocation"=w241, "Last Loaded File"=w242, "GUIName"="bob1tobun", "DIMControSet in"=w243, "SetValueInfo in"=w237, "NewVal"=w239) -> ()  [unwired: 14 in]
              }
            }
          }
          event Value Change {
            # "Update Last Loaded File"
            n164 = event-data() -> ("NewVal"=w247:T1)  [unwired: 1 in]
            n165 = control-ref of="Last Loaded File"() -> (w248:refnum<vi>)
            n166 = control-ref of="SetFileLocation"() -> (w249:refnum<vi>)
            n167 = call "LastLoadedFile.vi"("SetFileLocation"=w249, "Last Loaded File"=w248, "GUIName"="bob1tobun", "DIMControSet in"=w245, "SetValueInfo in"=w244, "NewVal"=w247) -> ()  [unwired: 14 in]
          }
          event Value Change {
            # "Find Monitor Value Index"
            # "Updating a Monitor Value"
            n168 = event-data() -> ("CtlRef"=w255:refnum<vi>, "NewVal"=w258:T2)  [unwired: 1 in, 4 out]
            n169 = Search 1D Array(1D array=w256, element=w255) -> (index of element=w254:i32)  [unwired: 1 in]
            n170 = Index Array(array=w253, index=w254) -> (element=w252:refnum<vi>)
            n171 = Not A Number/Path/Refnum?(number/path/refnum=w252) -> (NaN/Path/Refnum?=w251:bool)
            n172 = case "Indicator does not exists?" shown="False" w251 {
              tunnel: w258 -> [_ w265]
              tunnel: w252 -> [_ w259]
              frame True {
              }
              frame False {
                n173 = Unbundle By Name(w265) -> ("data"=w261:dbl, "no link"=w262:bool, "quality"=w264:i32)
                n174 = case shown="False" w262 {
                  tunnel: w264 -> [w268 _]
                  tunnel: [w267 UtilityLib.valueStatus."no info available" ("valueStatus")] -> w263
                  tunnel: w261 -> [w266 _]
                  tunnel: [w266 inf] -> w260
                  frame False {
                    n175 = call "CoreLib.quality 2 status.vi"("quality"=w268) -> ("valueStatus"=w267:T4)  [unwired: 18 in]
                  }
                  frame True {
                  }
                }
                n176 = property class="DigNum (strict)"(reference=w259, "Value"=w260) -> ()  [unwired: 1 in, 2 out]
                n177 = call "TextColor.vi"("valueStatus"=w263, "reference"=w259) -> ()  [unwired: 10 in]
              }
            }
          }
          event Value Change {
            n178 = event-data() -> ("CtlRef"=w274:refnum<vi>)  [unwired: 1 in, 5 out]
            n179 = property on="FileUpToDate" class="Bool (strict)"() -> ("Value"=w271:bool)  [unwired: 2 in, 2 out]
            n180 = call "FileUpToDate.vi"("FileUpToDate in"=w271, "DIMControSet out"=w273, "CtlRef"=w274) -> ("FileUpToDate out"=w272:bool)  [unwired: 16 in]
            n181 = property on="FileUpToDate" class="Bool (strict)"("Value"=w272) -> ()  [unwired: 2 in, 2 out]
          }
          event "BOB1DefY", "BOB1DefX", "WalLens", "BOB2DefY", "BOB2DefX", "Q90CylLens", "ISDefX", "Q90BOB3Lens", "Q90DefMain", "BOB2Q90Lens", "BOB3DefX", "BOB3DefY", "Q90PlanLens", "ISDefY", "Q90PlanDefY": Value Change {
            # "Find sub-panel index"
            # "opening or closing a sub-panel"
            n182 = event-data() -> ("CtlRef"=w277:refnum<vi>)  [unwired: 1 in, 3 out]
            n183 = Search 1D Array(1D array=w276, element=w277) -> (index of element=w282:i32)  [unwired: 1 in]
            n184 = Index Array(array=w283, index=w282) -> (element=w280:refnum<vi>)
            n185 = invoke class="Bool" method="Reinit To Default"(reference=w277) -> ()  [unwired: 2 in, 3 out]
            n186 = property class="VI"(reference=w280) -> ("Front Panel.Open"=w279:bool)  [unwired: 1 in, 2 out]
            n187 = case "Panel Already Open?" shown="True" w279 {
              tunnel: w280 -> [_ w287]
              tunnel: [w285 refnum<vi> refnum ("vi reference")] -> w278
              tunnel: w277 -> [w284 _]
              frame False {
                n188 = call "OpenPanel.vi"("CtlRef"=w284) -> ("vi reference"=w285:refnum<vi>)  [unwired: 2 in]
              }
              frame True {
                n189 = call "PanelClose.vi"("vi reference"=w287) -> ()
              }
            }
            n190 = Replace Array Subset(array=w283, new element=w278, index=w282) -> (w281:refnum<vi>[])
          }
          event "Close All Panels": Value Change {
            # "Close All Panels"
            n191 = event-data() -> ()  [unwired: 1 in, 6 out]
            n192 = case "Close Open Panels?" shown="True" "Close All Panels" {
              tunnel: w290 -> [w291 w293]
              tunnel: [w291 w292] -> w288
              frame False {
              }
              frame True {
                n193 = for "Close Open Panels" {
                  tunnel: w293 -> [w295] mode=indexing
                  tunnel: w293 -> [w294]
                  tunnel: [w294] -> w292
                  n194 = call "PanelClose.vi"("vi reference"=w295) -> ()
                }
              }
            }
          }
          event Timeout {
            # "Timeout"
            n195 = event-data() -> ()  [unwired: 1 in, 3 out]
          }
          event Panel Close? {
            n196 = event-data() -> ()  [unwired: 1 in, 4 out]
            n197 = stacked-sequence {
              tunnel: w300 -> [w307 _]
              tunnel: w299 -> [w305 _]
              tunnel: w298 -> [w304 _]
              tunnel: w297 -> [w303 _]
              frame #0 {
                # "Release DIM Services"
                n198 = for "Close Open Panels" {
                  tunnel: w307 -> [w317] mode=indexing
                  n199 = call "PanelClose.vi"("vi reference"=w317) -> ()
                }
                n200 = for "For Each Service" {
                  tunnel: w303 -> [w309] mode=indexing
                  n201 = Not A Number/Path/Refnum?(number/path/refnum=w309) -> (NaN/Path/Refnum?=w308:bool)
                  n202 = case "Not a Reference?" shown="False" w308 {
                    tunnel: w309 -> [w310 _]
                    frame False {
                      n203 = call "DimIndicators.dic_release_service.vi"("controlRef"=w310) -> ()  [unwired: 18 in, 1 out]
                    }
                    frame True {
                    }
                  }
                }
                n204 = for "For Each Service" {
                  tunnel: w304 -> [w312] mode=indexing
                  n205 = Not A Number/Path/Refnum?(number/path/refnum=w312) -> (NaN/Path/Refnum?=w311:bool)
                  n206 = case "Not a Reference?" shown="False" w311 {
                    tunnel: w312 -> [w313 _]
                    frame False {
                      n207 = call "DimIndicators.dic_release_service.vi"("controlRef"=w313) -> ()  [unwired: 18 in, 1 out]
                    }
                    frame True {
                    }
                  }
                }
                n208 = for "For Each Service" {
                  tunnel: w305 -> [w315] mode=indexing
                  n209 = Not A Number/Path/Refnum?(number/path/refnum=w315) -> (NaN/Path/Refnum?=w314:bool)
                  n210 = case "Not a Reference?" shown="False" w314 {
                    tunnel: w315 -> [w316 _]
                    frame False {
                      n211 = call "DimIndicators.dic_release_service.vi"("controlRef"=w316) -> ()  [unwired: 18 in, 1 out]
                    }
                    frame True {
                    }
                  }
                }
                n212 = control-ref of="SetFileLocation_Data"() -> (w302:refnum<vi>)
                n213 = control-ref of="Last Loaded File_Data"() -> (w306:refnum<vi>)
                n214 = call "DimIndicators.dic_release_service.vi"("controlRef"=w302) -> ()  [unwired: 18 in, 1 out]
                n215 = call "DimIndicators.dic_release_service.vi"("controlRef"=w306) -> ()  [unwired: 18 in, 1 out]
              }
              frame #1 {
                # "Close Front Panel"
                n216 = Current VI's Path() -> (path=w318:path)
                n217 = Open VI Reference(vi path=w318) -> (vi reference=w320:refnum<vi>, error out=w321:errorcluster)  [unwired: 5 in]
                n218 = property class="VI"(reference=w320, error in=w321, "Front Panel Window:Open"=FALSE) -> ()  [unwired: 2 out]
              }
            }
            n219 = event-data() -> ()  [unwired: 2 in, 1 out]
          }
        }
      }
    }
    frame #3 {
      n220 = stacked-sequence "Close Connections to DIM" {
        tunnel: w325 -> [w327 _ _]
        tunnel: w324 -> [w331 _ _]
        tunnel: w323 -> [w328 _ _]
        tunnel: w322 -> [w329 _ _]
        frame #0 {
          # "Release DIM Services"
          n221 = for "For Each Service" {
            tunnel: w329 -> [w339] mode=indexing
            n222 = Not A Number/Path/Refnum?(number/path/refnum=w339) -> (NaN/Path/Refnum?=w338:bool)
            n223 = case "Not a Reference?" shown="False" w338 {
              tunnel: w339 -> [w340 _]
              frame False {
                n224 = call "DimIndicators.dic_release_service.vi"("controlRef"=w340) -> ()  [unwired: 18 in, 1 out]
              }
              frame True {
              }
            }
          }
          n225 = for "For Each Service" {
            tunnel: w328 -> [w336] mode=indexing
            n226 = Not A Number/Path/Refnum?(number/path/refnum=w336) -> (NaN/Path/Refnum?=w335:bool)
            n227 = case "Not a Reference?" shown="False" w335 {
              tunnel: w336 -> [w337 _]
              frame False {
                n228 = call "DimIndicators.dic_release_service.vi"("controlRef"=w337) -> ()  [unwired: 18 in, 1 out]
              }
              frame True {
              }
            }
          }
          n229 = for "For Each Service" {
            tunnel: w327 -> [w333] mode=indexing
            n230 = Not A Number/Path/Refnum?(number/path/refnum=w333) -> (NaN/Path/Refnum?=w332:bool)
            n231 = case "Not a Reference?" shown="False" w332 {
              tunnel: w333 -> [w334 _]
              frame False {
                n232 = call "DimIndicators.dic_release_service.vi"("controlRef"=w334) -> ()  [unwired: 18 in, 1 out]
              }
              frame True {
              }
            }
          }
          n233 = control-ref of="Last Loaded File_Data"() -> (w330:refnum<vi>)
          n234 = control-ref of="SetFileLocation_Data"() -> (w326:refnum<vi>)
          n235 = for "Close Open Panels" {
            tunnel: w331 -> [w341] mode=indexing
            n236 = call "PanelClose.vi"("vi reference"=w341) -> ()
          }
          n237 = call "DimIndicators.dic_release_service.vi"("controlRef"=w330) -> ()  [unwired: 18 in, 1 out]
          n238 = call "DimIndicators.dic_release_service.vi"("controlRef"=w326) -> ()  [unwired: 18 in, 1 out]
        }
        frame #1 {
          # "Close Front Panel"
          n239 = Current VI's Path() -> (path=w345:path)
          n240 = Open VI Reference(vi path=w345) -> (vi reference=w343:refnum<vi>, error out=w342:errorcluster)  [unwired: 5 in]
          n241 = property class="VI"(reference=w343, error in=w342, "Front Panel Window:Open"=FALSE) -> ()  [unwired: 2 out]
        }
        frame #2 {
          # "Stop Panel"
          n242 = Stop(stop? (T)=TRUE) -> ()
        }
      }
    }
  }
  n243 = call "LVDimInterface.dim_operate.vi"("DNSNode"="lebit-balcony") -> ()  [unwired: 19 in]
